vi "ChipKit Light Show.vi"() -> ()   [LabVIEW 2011, in "LabVIEW Interface for ChipKit.lvlib"]
doc: "An Example that uses an ChipKit to control Tri Colored LEDs (or BlinkM's) based on wav audio data."
uses:
  vi.lib/LabVIEW Interface for ChipKit/LabVIEW Interface for ChipKit.lvlib
panel:
  in  "VISA resource name":refnum<visa-resource-name>
  out "Levels":dbl[](graph)
  out "Raw Sound Data":waveform(dbl)[](graph)
  in  "Cycle Colors":bool
  in  "Stop":bool
  in  "Samples Per Read":i32=3000
  in  "Start Position":i32
  in  ".wav File":path
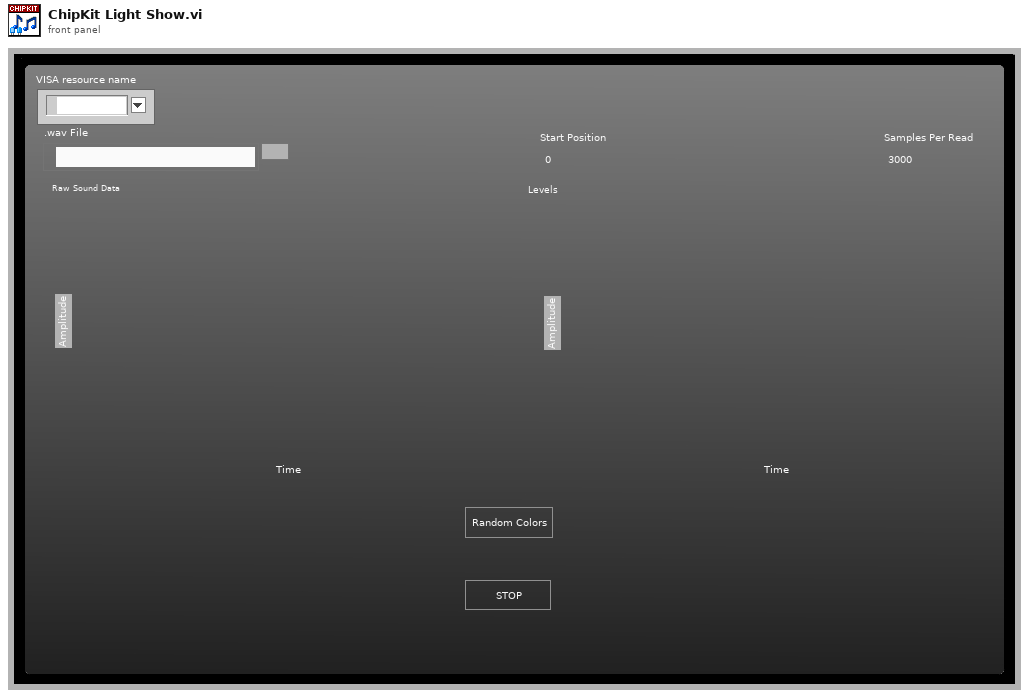
[diagram p1: front panel]
types:
  T1 = typedef "LabVIEW Interface for ChipKit.lvlib/Chipkit Resource.ctl" = cluster{"VISA resource":refnum<visa-resource-name>, "Board Type":T2, "Connection Type":enum8{"USB / Serial"}, "Bytes Per Packet (15)":u8}
  T2 = typedef "LabVIEW Interface for ChipKit.lvlib/Board Type.ctl" = enum16{"Arduino Uno", "Dimuelanove w/Atmega 328", "Mega 2560", "Chipkit Uno32", "Chipkit Max32"}
  T3 = typedef "LabVIEW Interface for ChipKit.lvlib/Chipkit Resource.ctl" = cluster{"COM Port":refnum<visa-resource-name>, "Board Type":T4, "Connection Type":T5, "Baud Rate (115200)":u32, "Bytes Per Packet (15)":u32}
  T4 = typedef "LabVIEW Interface for ChipKit.lvlib/Board Type.ctl" = enum16{"ChipKit uC32", "ChipKit Uno32", "ChipKit Max32"}
  T5 = typedef "LabVIEW Interface for ChipKit.lvlib/Connection Type.ctl" = enum8{"USB / Serial", "XBEE", "BlueSmirf (Bluetooth)"}
  T6 = typedef "Sound Output Task ID.ctl" = u32
  T7 = typedef "Sound File Refnum.ctl" = refnum<file>
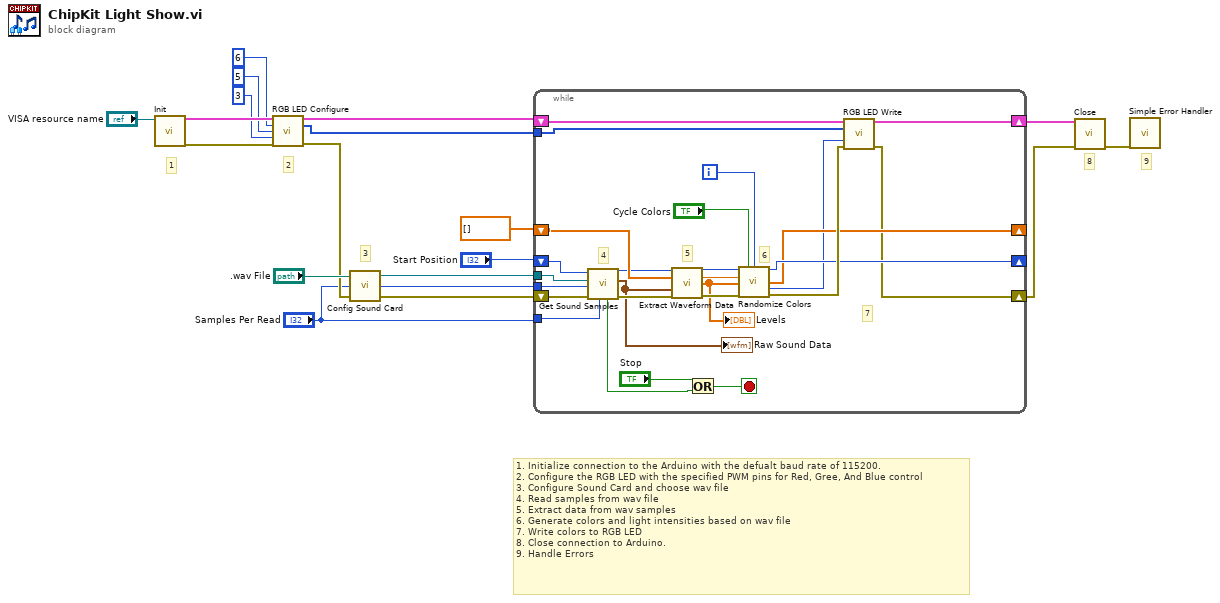
[diagram p0: block diagram]
diagram:
  # "9"
  # "8"
  # "3"
  # "2"
  # "1"
  # "1. Initialize connection to the Arduino with the defualt baud rate of 115200.\n2. Configure the RGB LED with the specified PWM pins for Red, Gree, And Blue control\n3. Configure Sound Card and choose wav file\n4. Read samples from wav file\n5. Extract data from wav samples\n6. Generate colors and light intensities based on wav file\n7. Write colors to RGB LED\n8. Close connection to Arduino.\n9. Handle Errors"
  n1 = call "Init.vi"("VISA resource"="VISA resource name") -> ("Arduino Resource"=w8:T1, "error out"=w7:errorcluster)  [unwired: 17 in]
  n2 = call "RGB LED Configure.vi"("Arduino Resource"=w8, "Red Pin"=6, "Green Pin"=5, "Blue Pin"=3, "error in"=w7) -> ("Arduino Resource"=w15:T3, "RGB LED Pins"=w2:u8[], "error out"=w12:errorcluster)  [unwired: 8 in]
  n3 = call "Config Sound Card.vi"("error in"=w12, "Samples Per Read"="Samples Per Read", "Song"=".wav File") -> ("error out"=w16:errorcluster, "task ID"=w19:T6, "sound file refnum"=w18:T7)
  n4 = while {
    shift-right: [w23] -> w14
    shift-left: w16 -> [w45]
    shift-right: [w35] -> _
    shift-left: "Start Position" -> [w41]
    shift-right: [w34] -> _
    shift-left: dbl[] [] -> [w32]
    shift-right: [w22] -> w6
    shift-left: w15 -> [w21]
    tunnel: "Samples Per Read" -> [w39]
    tunnel: w18 -> [w42]
    tunnel: w19 -> [w43]
    tunnel: w2 -> [w20]
    i -> [w44]
    stop <- w29 stop-if-true
    # "7"
    # "6"
    # "5"
    # "4"
    n5 = call "Get Sound Samples.vi"("error in"=w45, "task ID"=w43, "sound file refnum"=w42, "Sample Start Position"=w41, "Samples Per Read"=w39) -> ("end of file?"=w40:bool, "error out"=w38:errorcluster, "data"=w25:waveform(dbl)[], "Next Sample Start Position"=w30:i32)  [unwired: 2 in]
    "Raw Sound Data" <- w25
    n6 = call "Extract Waveform Data.vi"("Next Sample Start Position"=w30, "Previous Amplitudes"=w32, "data"=w25, "error in"=w38) -> ("Next Sample Start Position"=w31:i32, "Current Max"=w33:dbl, "Levels"=w24:dbl[], "error out"=w37:errorcluster)  [unwired: 8 in]
    "Levels" <- w24
    n7 = Or(x="Stop", y=w40) -> (x .or. y?=w29:bool)
    n8 = call "Randomize Colors.vi"("Next Sample Start Position"=w31, "Cycle Colors?"="Cycle Colors", "Iteration"=w44, "Current Max"=w33, "Levels"=w24, "error in"=w37) -> ("Next Sample Start Position"=w35:i32, "Levels"=w34:dbl[], "Color"=w28:u32, "error out"=w36:errorcluster)  [unwired: 6 in]
    n9 = call "RGB LED Write.vi"("Arduino Resource"=w21, "RGB LED Pins"=w20, "Color"=w28, "error in"=w36) -> ("Arduino Resource"=w22:T3, "error out"=w23:errorcluster)  [unwired: 9 in, 1 out]
  }
  n10 = call "Close.vi"("Arduino Resource"=w6, "error in"=w14) -> ("error out"=w13:errorcluster)  [unwired: 13 in]
  n11 = call <vilib>:"Simple Error Handler.vi"("error in (no error)"=w13) -> ()  [unwired: 4 in, 5 out]
